vi "B Sweep Rabi measurements.vi"() -> ()   [LabVIEW 2012]
uses:
  <vilib>/Utility/file.llb/Read From Spreadsheet File (DBL).vi
  <vilib>/Utility/file.llb/Write To Spreadsheet File (DBL).vi
  <vilib>/express/express arith-compare/Formula/XNode/ExpressFormulaBlockNode.xnode
panel:
  out "ODMR freq":ext
  in  "MW width Min":dbl=5e-08
  in  "MW width Max":dbl=5e-07
  in  "MW width step size":dbl=2e-09
  in  "MW Delay":dbl
  in  "ODMR res file":path
  in  "GPIB Address":string="20"
  in  "band (1-26.5 GHz:20)":i32(ring)=2
  in  "resolution (1 Hz:1)":i32(ring)=1 items=["0.1 Hz", "1 Hz", "10 Hz", "100 Hz", "1 KHz", "10 KHz", "100 KHz", "1 MHz", "10 MHz", "100 MHz", "1 GHz"]
  in  "RS232 settings":cluster{"Portnumber":i32, "Baudrate":u16}={"Portnumber"=12, "Baudrate"=5} {"Portnumber" items=["COM1", "COM2", "COM3", "COM4", "COM5", "COM6", "COM7", "COM8", "COM9", "COM10", "COM11", "COM12", "COM13", "COM14", "COM15", "COM16", "COM17", "COM18", "COM19", "COM20", "COM21", "COM22", "COM23", "COM24", "COM25", "COM26", "COM27", "COM28", "COM29", "COM30"]; "Baudrate" items=["9600", "14400", "19200", "38400", "57600", "115200"]}
  in  "Z Pos":dbl=77.35
  in  "Y pos":dbl=9.0
  in  "X Pos":dbl=41.0
  in  "Y Parameters":T1={"Number of Y Steps"=200, "Max Y (V)"=2.0, "Min Y (V)"=-2.0}
  in  "X":T2={"Number of X Steps"=200, "Max X (V)"=2.0, "Min X (V)"=-2.0}
  out "Tracking Loop":dbl=6.0
  in  "N Loop":i32=25000
  in  "ref?":bool=TRUE
  in  "Sig/Ref pause":dbl=3e-07
  in  "APD signal width":dbl=3e-07
  in  "AOM Pulse length":dbl=2.5e-06
  in  "Signal delay":dbl=1.16e-06
  in  "AOM Rest time":dbl=2e-08
  in  "Path to spinapi.dll":path=path "C:/SpinCore/SpinAPI/dll/spinapi64.dll"
  in  "Scan Interval (sec)":dbl=2.0
  in  "Collection Time (sec)":dbl=3.0
  in  "File Path Control":path
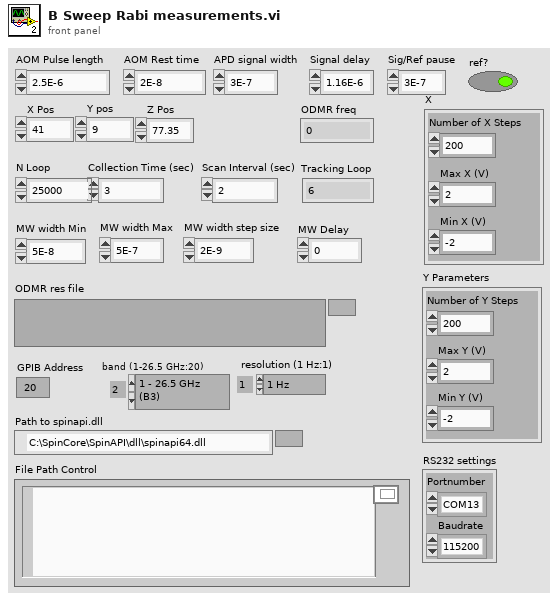
[diagram p1: front panel]
types:
  T1 = cluster{"Number of Y Steps":i32, "Max Y (V)":dbl, "Min Y (V)":dbl}
  T2 = cluster{"Number of X Steps":i32, "Max X (V)":dbl, "Min X (V)":dbl}
  T3 = enum16{"Stop", "ODMR", "Track", "EPR", "Load Pulse Sequence"}
  T4 = enum16{"Pulse Program", "Frequency Registers", "TX Phase Registers", "RX Phase Registers"}
  T5 = cluster{"source lock":bool, "lock frequency (Hz)":ext, "coarse tune":bool}
  T6 = cluster{"GPIB address 2":string, "resolution (10 Hz:2) 2":i32, "band (1-26.5:2) 2":i32, "Freq max":ext, "Start Voltage":dbl, "Voltage Step":dbl, "rate":dbl, "samples per channel":i32}
  T7 = cluster{"RS232 settings":cluster{"Portnumber":i32, "Baudrate":u16}, "X Parameters":cluster{"Number of X Steps":i32, "Max X (V)":dbl, "Min X (V)":dbl}, "Y Parameters":cluster{"Number of Y Steps":i32, "Max Y (V)":dbl, "Min Y (V)":dbl}, "X Pos":dbl, "Y Pos":dbl, "Z Pos":dbl, "Tracking interval":dbl}
  T8 = cluster{"Instruct Data":i32, "Op Code":i32, "Flags":bool[], "Comments":string, "Time (s)":dbl}
  T9 = cluster{"Instruct Data":i32, "Op Code":i32, "Flags":bool[], "Comments":string, "Time (s)":dbl}[]
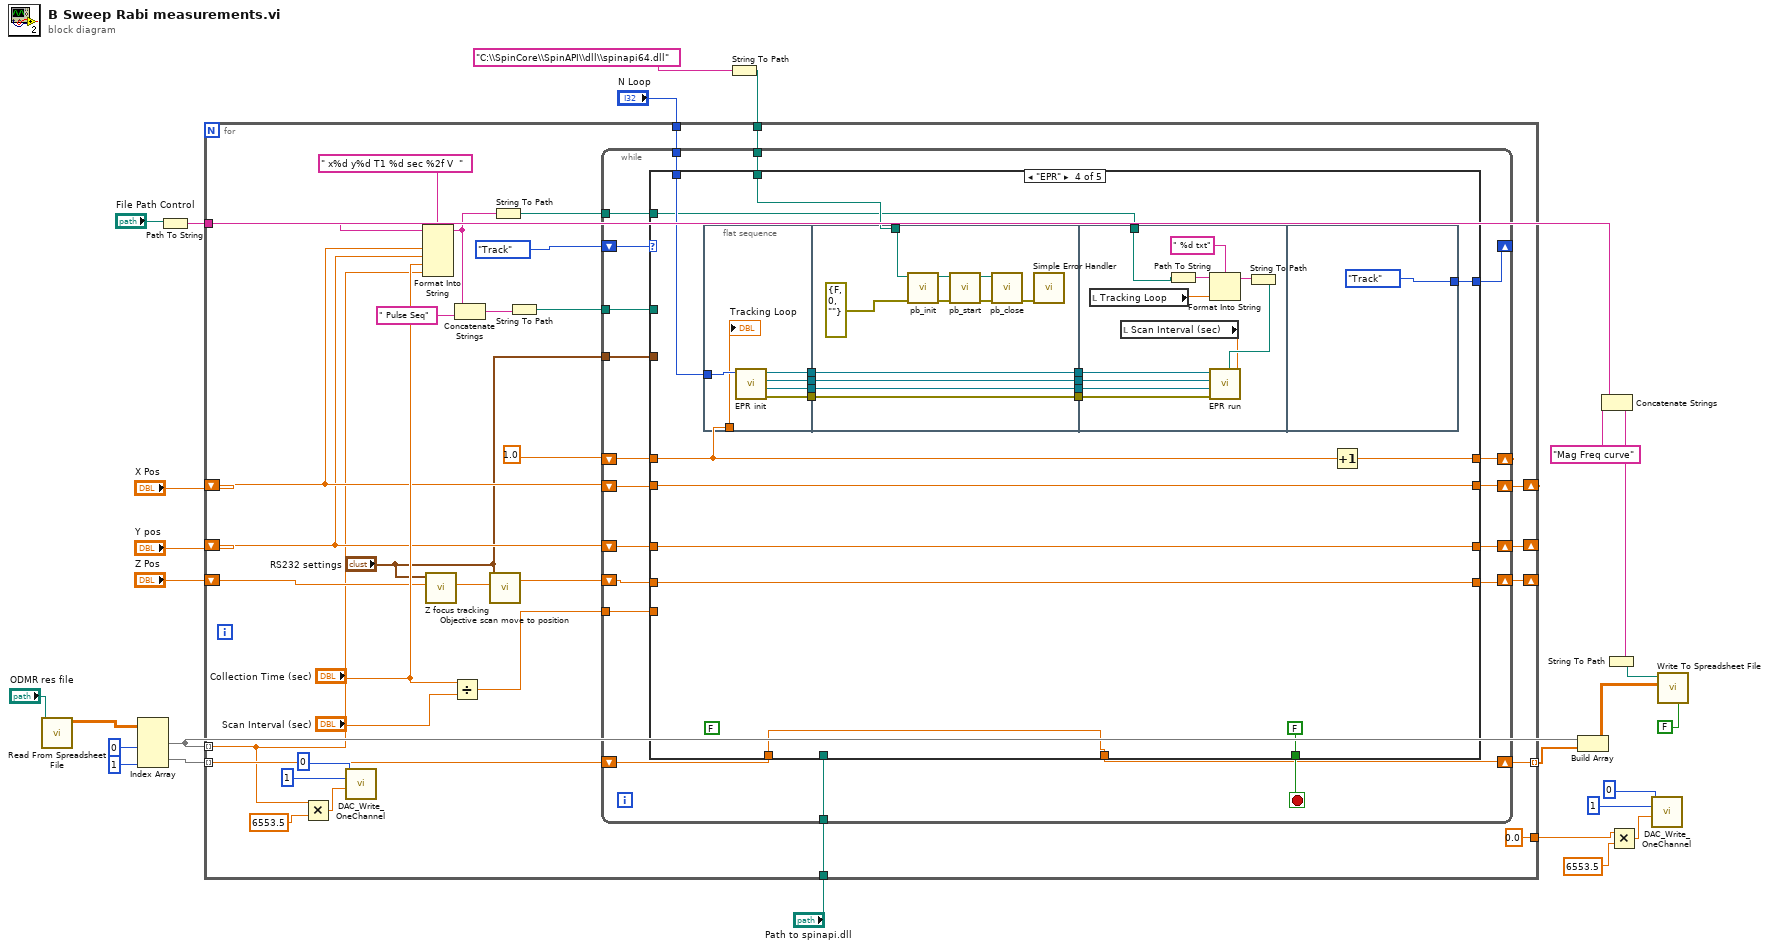
[diagram p0: block diagram]
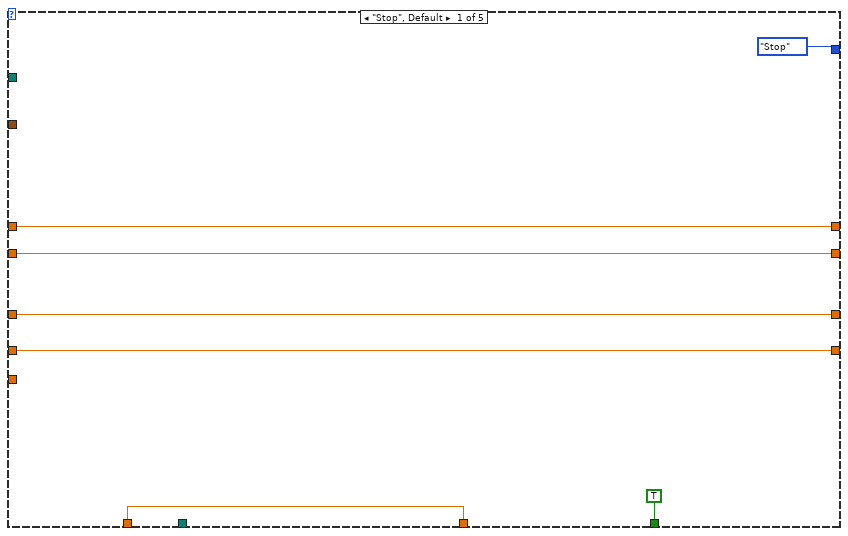
[diagram p2: hidden frame]
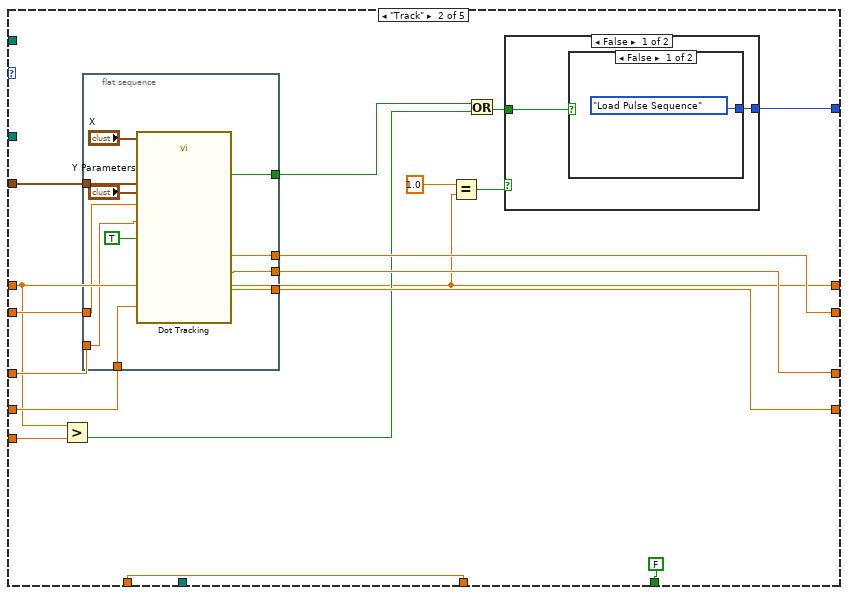
[diagram p3: hidden frame]
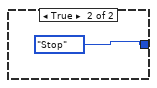
[diagram p4: hidden frame]
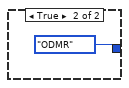
[diagram p5: hidden frame]
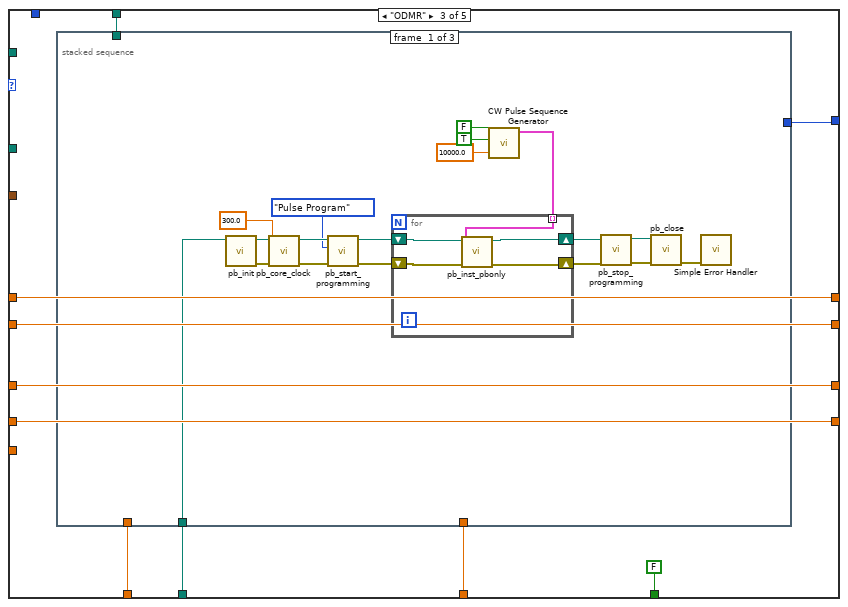
[diagram p6: hidden frame]
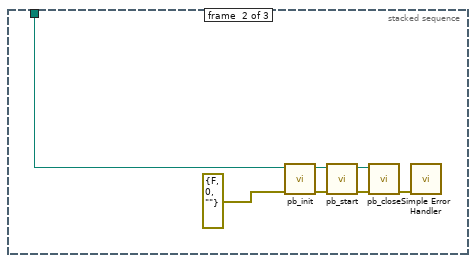
[diagram p7: hidden frame]
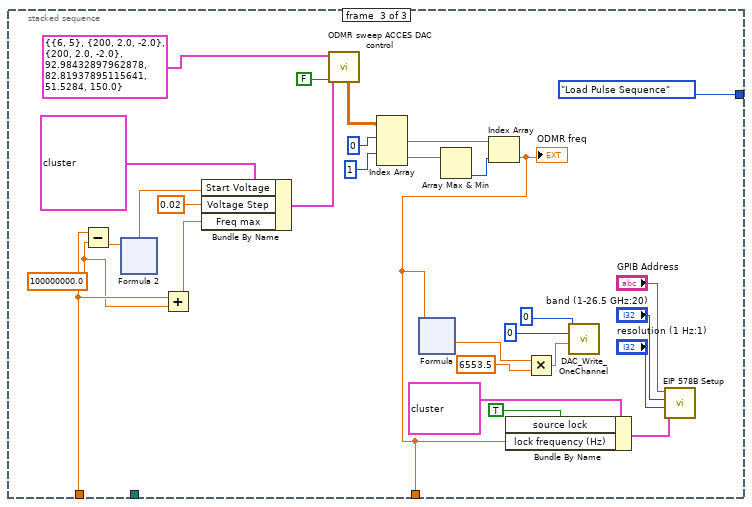
[diagram p8: hidden frame]
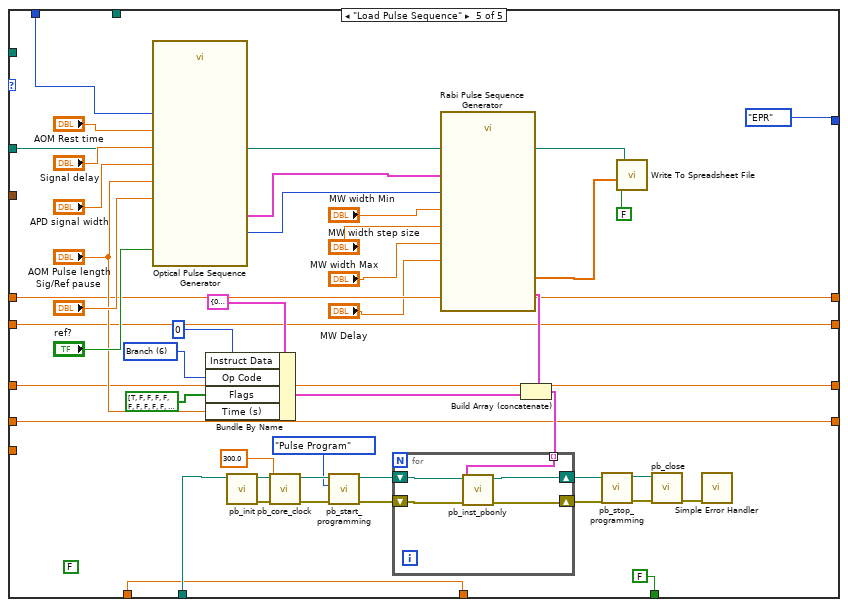
[diagram p9: hidden frame]
diagram:
  n1 = call-poly <vilib>:"Read From Spreadsheet File.vi"("file path (dialog if empty)"="ODMR res file") -> ("all rows"=w12:dbl[][])  [unwired: 6 in, 4 out]
  n2 = Index Array(array=w12, index (col) #1=0 ("disabled index (col)"), index (col) #2=1 ("index (col)")) -> (element #1=w7:dbl[], element #2=w10:dbl[])  [unwired: 2 in]
  n3 = Path To String(path="File Path Control") -> (string=w4:string)
  n4 = String To Path(string="C:\\SpinCore\\SpinAPI\\dll\\spinapi64.dll") -> (path=w24:path)
  n5 = for {
    shift-right: [w54] -> _
    shift-left: "X Pos" -> [w39]
    shift-right: [w53] -> _
    shift-left: "Y pos" -> [w38]
    tunnel: w4 -> [w58]
    tunnel: w24 -> [w55]
    tunnel: "N Loop" -> [w52]
    shift-right: [w43] -> _
    shift-left: "Z Pos" -> [w41]
    tunnel: [0.0 ("x")] -> w15
    tunnel: w7 -> [w29] mode=indexing
    tunnel: w10 -> [w30] mode=indexing
    tunnel: "Path to spinapi.dll" -> [w28]
    tunnel: [w27] -> w8 mode=indexing
    n6 = Multiply(x=w29, y=6553.5) -> (x*y=w35:dbl)
    n7 = call "DAC_Write_OneChannel.vi"("Value"=w35, "Channel"=u16 1, "DeviceIndex"=u64 0) -> ()  [unwired: 7 in, 2 out]
    n8 = Format Into String(format string=" x%d y%d T1 %d sec %2f V  ", initial string=w58, w39, w38, "Collection Time (sec)", w29) -> (resulting string=w51:string)  [unwired: 1 in, 1 out]
    n9 = call "Z focus tracking.vi"("Position"=w41, "RS232 settings"="RS232 settings") -> ("center"=w42:dbl)  [unwired: 6 in, 2 out]
    n10 = Divide(x="Collection Time (sec)", y="Scan Interval (sec)") -> (x/y=w45:dbl)
    n11 = Concatenate Strings(w51, " Pulse Seq" ("string")) -> (w49:string)
    n12 = call "Objective scan move to position.vi"("Z position"=w42, "RS232 settings"="RS232 settings") -> ("Z Position 2"=w40:dbl)  [unwired: 9 in]
    n13 = String To Path(string=w51) -> (path=w50:path)
    n14 = String To Path(string=w49) -> (path=w48:path)
    n15 = while {
      tunnel: w55 -> [w78]
      shift-right: [w76] -> w54
      shift-left: w39 -> [w75]
      shift-right: [w77] -> w53
      shift-left: w38 -> [w74]
      tunnel: w52 -> [w72]
      tunnel: w50 -> [w71]
      tunnel: w48 -> [w70]
      shift-right: [w68] -> _
      shift-left: 1.0 -> [w69]
      tunnel: w45 -> [w67]
      shift-right: [w65] -> w43
      shift-left: w40 -> [w66]
      tunnel: "RS232 settings" -> [w64]
      shift-right: [w62] -> _
      shift-left: T3."Track" -> [w63]
      tunnel: w28 -> [w60]
      shift-right: [w59] -> w27
      shift-left: w30 -> [w61]
      stop <- w73 stop-if-true
      n16 = case shown="\"EPR\"" w63 {
        tunnel: w78 -> [_ _ w120 w214 _]
        tunnel: [w83 w96 w126 w211 w261] -> w76
        tunnel: [w82 w95 w127 w207 w260] -> w77
        tunnel: w75 -> [w83 w93 w126 w211 w261]
        tunnel: w74 -> [w82 w92 w127 w207 w260]
        tunnel: [T3."Stop" w101 w123 w208 T3."EPR"] -> w62
        tunnel: [TRUE FALSE FALSE FALSE FALSE] -> w73
        tunnel: w72 -> [_ _ _ w213 w264]
        tunnel: w71 -> [_ _ _ w212 _]
        tunnel: w70 -> [_ _ _ _ w263]
        tunnel: w69 -> [w84 w88 w125 w206 w262]
        tunnel: [w84 w88 w125 w209 w262] -> w68
        tunnel: w67 -> [_ w99 _ _ _]
        tunnel: w66 -> [w81 w97 w128 w205 w259]
        tunnel: [w81 w94 w128 w205 w259] -> w65
        tunnel: w64 -> [_ w91 _ _ _]
        tunnel: w61 -> [w79 w86 w124 w204 w252]
        tunnel: w60 -> [_ _ w121 _ w253]
        tunnel: [w79 w86 w119 w204 w252] -> w59
        frame "Stop", Default {
        }
        frame "Track" {
          n17 = Greater?(x=w88, y=w99) -> (0:w90:bool)
          n18 = flat-sequence {
            tunnel: [w118] -> w96
            tunnel: [w117] -> w95
            tunnel: [w115] -> w102
            tunnel: w97 -> [w112]
            tunnel: [w111] -> w94
            tunnel: w93 -> [w110]
            tunnel: w92 -> [w109]
            tunnel: w91 -> [w108]
            frame #0 {
              n19 = call "Dot Tracking.vi"("X"="X", "Y Parameters"="Y Parameters", "RS232 settings"=w108, "X Pos"=w110, "Y pos"=w109, "Z Pos"=w112, "Z-track?"=TRUE) -> ("X Position"=w118:dbl, "Y Position"=w117:dbl, "Z Position"=w111:dbl, "Gave up?"=w115:bool)  [unwired: 2 in, 3 out]
            }
          }
          n20 = Equal?(x=1.0, y=w88) -> (x = y?=w89:bool)
          n21 = Or(x=w102, y=w90) -> (x .or. y?=w98:bool)
          n22 = case shown="False" w89 {
            tunnel: [w104 T3."ODMR"] -> w101
            tunnel: w98 -> [w103 _]
            frame False {
              n23 = case shown="False" w103 {
                tunnel: [T3."Load Pulse Sequence" T3."Stop"] -> w104
                frame False {
                }
                frame True {
                }
              }
            }
            frame True {
            }
          }
        }
        frame "ODMR" {
          n24 = stacked-sequence {
            tunnel: w124 -> [_ _ w182]
            tunnel: [_ _ T3."Load Pulse Sequence"] -> w123
            tunnel: w121 -> [w129 _ _]
            tunnel: w120 -> [_ w152 _]
            tunnel: [_ _ w161] -> w119
            frame #0 {
              n25 = call "pb_init.vi"("path in"=w129) -> ("error out"=w139:errorcluster, "path out"=w137:path)  [unwired: 3 in, 6 out]
              n26 = call "pb_core_clock.vi"("error in (no error)"=w139, "clock_freq (MHz)"=300.0, "path in"=w137) -> ("error out"=w140:errorcluster, "path out"=w138:path)  [unwired: 7 in]
              n27 = call "pb_start_programming.vi"("error in (no error)"=w140, "Device"=T4."Pulse Program", "path in"=w138) -> ("error out"=w143:errorcluster, "path out"=w142:path)  [unwired: 1 in, 6 out]
              n28 = call "CW Pulse Sequence Generator.vi"("Pulse Laser"=FALSE, "Pulse MW"=TRUE, "Rate (Hz)"=10000.0) -> ("Pulse Sequence Out"=w133:T9)  [unwired: 7 in]
              n29 = for {
                shift-right: [w149] -> w144
                shift-left: w142 -> [w151]
                shift-right: [w148] -> w145
                shift-left: w143 -> [w150]
                tunnel: w133 -> [w147] mode=indexing
                n30 = call "pb_inst_pbonly.vi"("error in (no error)"=w150, "PB Instruction"=w147, "path in"=w151) -> ("error out"=w148:errorcluster, "path out"=w149:path)  [unwired: 2 in, 5 out]
              }
              n31 = call "pb_stop_programming.vi"("error in (no error)"=w145, "path in"=w144) -> ("error out"=w136:errorcluster, "path out"=w135:path)  [unwired: 1 in, 7 out]
              n32 = call "pb_close.vi"("error in (no error)"=w136, "path in"=w135) -> ("error out"=w146:errorcluster)  [unwired: 9 out]
              n33 = call <vilib>:"Simple Error Handler.vi"("error in (no error)"=w146) -> ()  [unwired: 1 in, 8 out]
            }
            frame #1 {
              n34 = call "pb_init.vi"("error in (no error)"=errorcluster {"status"=FALSE, "code"=0, "source"=""}, "path in"=w152) -> ("error out"=w156:errorcluster, "path out"=w154:path)  [unwired: 1 in, 7 out]
              n35 = call "pb_start.vi"("error in (no error)"=w156, "path in"=w154) -> ("error out"=w157:errorcluster, "path out"=w153:path)  [unwired: 1 in, 7 out]
              n36 = call "pb_close.vi"("error in (no error)"=w157, "path in"=w153) -> ("error out"=w158:errorcluster)  [unwired: 9 out]
              n37 = call <vilib>:"Simple Error Handler.vi"("error in (no error)"=w158) -> ()  [unwired: 1 in, 8 out]
            }
            frame #2 {
              w181 = 100000000.0 ("y")
              n38 = Subtract(x=w182, y=w181) -> (x-y=w183:ext)
              n39 = xnode "Formula 2"("X1"=w183) -> ("Result"=w184:ext)  [unwired: 1 in, 1 out]
              n40 = Add(x=w182, y=w181) -> (x+y=w180:ext)
              n41 = Bundle By Name(cluster=T6 {"GPIB address 2"="19", "resolution (10 Hz:2) 2"=2, "band (1-26.5:2) 2"=2, "Freq max"=4000000000.0, "Start Voltage"=0.0, "Voltage Step"=0.02, "rate"=100.0, "samples per channel"=200} ("Freq Sweep Cluster"), "Start Voltage"=w184, "Voltage Step"=0.02, "Freq max"=w180) -> (w185:T6)
              n42 = call "ODMR sweep ACCES DAC control.vi"("Save?"=FALSE, "Freq Sweep Cluster"=w185, "Dot Tracking Cluster"=T7 {"RS232 settings"={"Portnumber"=6, "Baudrate"=5}, "X Parameters"={"Number of X Steps"=200, "Max X (V)"=2.0, "Min X (V)"=-2.0}, "Y Parameters"={"Number of Y Steps"=200, "Max Y (V)"=2.0, "Min Y (V)"=-2.0}, "X Pos"=92.98432897962878, "Y Pos"=82.81937895115641, "Z Pos"=51.5284, "Tracking interval"=150.0}) -> ("appended array"=w177:ext[][])  [unwired: 4 in, 4 out]
              n43 = Index Array(array=w177, index (row) #1=0 ("disabled index (col)"), index (row) #2=1 ("index (col)")) -> (element #1=w175:ext[], element #2=w176:ext[])  [unwired: 2 in]
              n44 = Array Max & Min(array=w176) -> (min index (indices)=w174:i32)  [unwired: 3 out]
              n45 = Index Array(array=w175, index=w174) -> (element=w161:ext)
              "ODMR freq" <- w161
              n46 = xnode "Formula"("X1"=w161) -> ("Result"=w169:ext)  [unwired: 1 in, 1 out]
              n47 = Bundle By Name(cluster=T5 {"source lock"=TRUE, "lock frequency (Hz)"=1000000000.0, "coarse tune"=TRUE} ("source locking"), "source lock"=TRUE, "lock frequency (Hz)"=w161) -> (w164:T5)
              n48 = Multiply(x=w169, y=6553.5) -> (x*y=w172:ext)
              n49 = call "DAC_Write_OneChannel.vi"("Value"=w172, "Channel"=u16 0, "DeviceIndex"=u64 0) -> ()  [unwired: 7 in, 2 out]
              n50 = call "EIP 578B Setup.vi"("GPIB Address"="GPIB Address", "band (1-26.5 GHz:20)"="band (1-26.5 GHz:20)", "resolution (1 Hz:1)"="resolution (1 Hz:1)", "source locking"=w164) -> ()  [unwired: 2 in, 2 out]
            }
          }
        }
        frame "EPR" {
          (unwired) FALSE
          n51 = flat-sequence {
            tunnel: [w228] -> w222
            tunnel: [w227] -> w221
            tunnel: [w226] -> w220
            tunnel: [w225] -> w219
            tunnel: w213 -> [w224]
            tunnel: w206 -> [w223]
            tunnel: [w233] -> w218
            tunnel: w222 -> [w233]
            tunnel: [w232] -> w217
            tunnel: w221 -> [w232]
            tunnel: [w231] -> w216
            tunnel: w220 -> [w231]
            tunnel: [w230] -> w215
            tunnel: w219 -> [w230]
            tunnel: w214 -> [w229]
            tunnel: w218 -> [w244]
            tunnel: w217 -> [w243]
            tunnel: w216 -> [w242]
            tunnel: w215 -> [w241]
            tunnel: w212 -> [w240]
            tunnel: [T3."Track"] -> w208
            frame #0 {
              n52 = call "EPR init.vi"("N loops"=w224) -> ("error out"=w225:errorcluster, "ref task out"=w226:refnum<k21>, "sig task out"=w227:refnum<k21>, "clock task out"=w228:refnum<k21>)  [unwired: 7 in]
              "Tracking Loop" <- w223
            }
            frame #1 {
              n53 = call "pb_init.vi"("error in (no error)"=errorcluster {"status"=FALSE, "code"=0, "source"=""}, "path in"=w229) -> ("error out"=w237:errorcluster, "path out"=w235:path)  [unwired: 1 in, 7 out]
              n54 = call "pb_start.vi"("error in (no error)"=w237, "path in"=w235) -> ("error out"=w238:errorcluster, "path out"=w234:path)  [unwired: 1 in, 7 out]
              n55 = call "pb_close.vi"("error in (no error)"=w238, "path in"=w234) -> ("error out"=w239:errorcluster)  [unwired: 9 out]
              n56 = call <vilib>:"Simple Error Handler.vi"("error in (no error)"=w239) -> ()  [unwired: 1 in, 8 out]
            }
            frame #2 {
              n57 = local read "Tracking Loop"() -> (w247:dbl)
              n58 = local read "Scan Interval (sec)"() -> (w245:dbl)
              n59 = Path To String(path=w240) -> (string=w249:string)
              n60 = Format Into String(format string=" %d txt", initial string=w249, w247) -> (resulting string=w248:string)  [unwired: 1 in, 1 out]
              n61 = String To Path(string=w248) -> (path=w246:path)
              n62 = call "EPR run.vi"("control task in"=w244, "sig task in"=w243, "ref task in"=w242, "error in"=w241, "file path (dialog if empty)"=w246, "Measurement Interval"=w245) -> ()  [unwired: 4 in]
            }
            frame #3 {
            }
          }
          n63 = Increment(x=w206) -> (x+1=w209:dbl)
        }
        frame "Load Pulse Sequence" {
          (unwired) FALSE
          w289 = 6 items=["Continue", "Stop", "Loop", "End Loop", "JSR", "RTS", "Branch", "Long Delay", "Wait"] ("Op Code")
          n64 = call "Optical Pulse Sequence Generator.vi"("ref?"="ref?", "N Loop"=w264, "Sig/Ref pause"="Sig/Ref pause", "AOM Rest time"="AOM Rest time", "Signal delay"="Signal delay", "APD signal width"="APD signal width", "AOM Pulse length"="AOM Pulse length") -> ("Array"=w271:T9, "No. Instructions"=w270:i32)  [unwired: 3 in]
          n65 = Bundle By Name(cluster=T8 {"Instruct Data"=0, "Op Code"=0, "Flags"=[FALSE, FALSE, FALSE, FALSE, FALSE, FALSE, FALSE, FALSE, FALSE, FALSE, FALSE, FALSE, FALSE, FALSE, FALSE, FALSE, FALSE, FALSE, FALSE, FALSE, FALSE, TRUE, TRUE, TRUE], "Comments"="", "Time (s)"=0.01} ("PB Inst 2"), "Instruct Data"=0, "Op Code"=w289, "Flags"=bool[] [TRUE, FALSE, FALSE, FALSE, FALSE, FALSE, FALSE, FALSE, FALSE, FALSE, FALSE, FALSE, FALSE, FALSE, FALSE, FALSE, FALSE, FALSE, FALSE, FALSE, FALSE, TRUE, TRUE, TRUE], "Time (s)"="AOM Pulse length") -> (w268:T8)
          n66 = call "pb_init.vi"("path in"=w253) -> ("error out"=w279:errorcluster, "path out"=w277:path)  [unwired: 3 in, 6 out]
          n67 = call "pb_core_clock.vi"("error in (no error)"=w279, "clock_freq (MHz)"=300.0, "path in"=w277) -> ("error out"=w280:errorcluster, "path out"=w278:path)  [unwired: 7 in]
          n68 = call "pb_start_programming.vi"("error in (no error)"=w280, "Device"=T4."Pulse Program", "path in"=w278) -> ("error out"=w283:errorcluster, "path out"=w282:path)  [unwired: 1 in, 6 out]
          n69 = call "Rabi Pulse Sequence Generator.vi"("Optical Pulse"=w271, "No. Instructions"=w270, "MW Delay"="MW Delay", "MW width step size"="MW width step size", "MW width Max"="MW width Max", "MW width Min"="MW width Min") -> ("Pulse Width"=w266:dbl[], "Pulse Sequence Out"=w269:T9)  [unwired: 4 in]
          n70 = Build Array (concatenate)(w269, w268) -> (w267:T9)
          n71 = for {
            shift-right: [w298] -> w284
            shift-left: w282 -> [w300]
            shift-right: [w297] -> w285
            shift-left: w283 -> [w299]
            tunnel: w267 -> [w296] mode=indexing
            n72 = call "pb_inst_pbonly.vi"("error in (no error)"=w299, "PB Instruction"=w296, "path in"=w300) -> ("error out"=w297:errorcluster, "path out"=w298:path)  [unwired: 2 in, 5 out]
          }
          n73 = call "pb_stop_programming.vi"("error in (no error)"=w285, "path in"=w284) -> ("error out"=w276:errorcluster, "path out"=w275:path)  [unwired: 1 in, 7 out]
          n74 = call-poly <vilib>:"Write To Spreadsheet File.vi"("transpose? (no:F)"=FALSE, "1D data"=w266, "file path (dialog if empty)"=w263) -> ()  [unwired: 5 in, 1 out]
          n75 = call "pb_close.vi"("error in (no error)"=w276, "path in"=w275) -> ("error out"=w286:errorcluster)  [unwired: 9 out]
          n76 = call <vilib>:"Simple Error Handler.vi"("error in (no error)"=w286) -> ()  [unwired: 1 in, 8 out]
        }
      }
    }
  }
  n77 = Build Array(w7, w8) -> (w5:ext[][])
  n78 = Concatenate Strings(w4, "Mag Freq curve" ("string")) -> (w2:string)
  n79 = String To Path(string=w2) -> (path=w3:path)
  n80 = Multiply(x=w15, y=6553.5) -> (x*y=w18:dbl)
  n81 = call "DAC_Write_OneChannel.vi"("Value"=w18, "Channel"=u16 1, "DeviceIndex"=u64 0) -> ()  [unwired: 7 in, 2 out]
  n82 = call-poly <vilib>:"Write To Spreadsheet File.vi"("transpose? (no:F)"=FALSE, "2D data"=w5, "file path (dialog if empty)"=w3) -> ()  [unwired: 5 in, 1 out]
